vi "FuzzyEx Tanks with PI control.vi"() -> ()   [LabVIEW 2023]
doc: "This example simulates a two-tank system with a fuzzy controller. The system is two tanks of water with a small orifice between the tanks at the bottom of both (height = 0 m). The second tank has another small orifice at the tank bottom that empties into a reservoir at a lower height than the two tanks. The initial properties of the tanks and orifices are shown on the front panel controls below each tank.\n\nThe goal of the simulation is to control the height of tank 2 to the user-specified height setpoint. The control value is the flow rate into tank 1. Therefore, this system is a second-order control system.\n\nThe tanks.fs file represents a fuzzy system with two inputs and one output. The inputs are the height error of tank 2 and the rate of change in height of tank 2. The controller output is the rate of change in flow rate into tank 1."
uses:
  <vilib>/addons/Fuzzy Logic/TypeDefs/FL System.ctl
  <vilib>/addons/Fuzzy Logic/TypeDefs/FL Variable.ctl
  <vilib>/addons/Fuzzy Logic/TypeDefs/FL Membership Function.ctl
  <vilib>/addons/Fuzzy Logic/TypeDefs/FL Membership Function Shape.ctl
  <vilib>/addons/Fuzzy Logic/TypeDefs/FL Rule.ctl
  <vilib>/addons/Fuzzy Logic/TypeDefs/FL Antecedent.ctl
  <vilib>/addons/Fuzzy Logic/TypeDefs/FL Modifier.ctl
  <vilib>/addons/Fuzzy Logic/TypeDefs/FL Antecedent Connective.ctl
  <vilib>/addons/Fuzzy Logic/TypeDefs/FL Consequent.ctl
  <vilib>/addons/Fuzzy Logic/TypeDefs/FL Consequent Implication.ctl
  <vilib>/addons/Fuzzy Logic/TypeDefs/FL Defuzzification.ctl
  <vilib>/addons/Fuzzy Logic/TypeDefs/FL Interpolating polynomials.ctl
  <vilib>/addons/Fuzzy Logic/FL Fuzzy Controller (MISO).vi
  <vilib>/addons/Fuzzy Logic/NI_Fuzzy_Logic_API.lvlib
panel:
  out "fuzzy system out":T1={"input variables"=[{"name"="dH/dT Tank 2", "range"=[-0.01, 0.01, -0.01, 0.01], "MFs"=[{"name"="Fast neg", "shape"=1, "points"=[-0.01, -0.01, -0.006666666666666668, -0.0026666666666666683], "color"=16711680, "user-defined shape index"=0}, {"name"="Slow neg", "shape"=0, "points"=[-0.006666666666666668, -0.0026666666666666683, 0.0], "color"=3342438, "user-defined shape index"=0}, {"name"="Zero", "shape"=0, "points"=[-0.0026666666666666683, 0.0, 0.0026666666666666705], "color"=255, "user-defined shape index"=0}, {"name"="Slow pos", "shape"=0, "points"=[0.0, 0.0026666666666666705, 0.006666666666666665], "color"=16724991, "user-defined shape index"=0}, {"name"="Fast pos", "shape"=1, "points"=[0.0026666666666666705, 0.006666666666666665, 0.01, 0.01], "color"=26214, "user-defined shape index"=0}]}, {"name"="Tank 2 error", "range"=[-0.5, 0.5, -0.5, 0.5], "MFs"=[{"name"="Lg neg", "shape"=1, "points"=[-0.5, -0.5, -0.3, -0.09999999999999998], "color"=16711680, "user-defined shape index"=0}, {"name"="Sm neg", "shape"=0, "points"=[-0.3, -0.09999999999999998, 0.0], "color"=3342438, "user-defined shape index"=0}, {"name"="None", "shape"=0, "points"=[-0.09999999999999998, 0.0, 0.09999999999999998], "color"=16724991, "user-defined shape index"=0}, {"name"="Sm pos", "shape"=0, "points"=[0.0, 0.09999999999999998, 0.30000000000000004], "color"=255, "user-defined shape index"=0}, {"name"="Lg pos", "shape"=1, "points"=[0.09999999999999998, 0.30000000000000004, 0.5, 0.5], "color"=26214, "user-defined shape index"=0}]}], "output variables"=[{"name"="Flow change", "range"=[-0.05, 0.05, -0.05, 0.05], "MFs"=[{"name"="Lg neg", "shape"=0, "points"=[-0.05, -0.05, -0.029999999999999995], "color"=16711680, "user-defined shape index"=0}, {"name"="Med neg", "shape"=0, "points"=[-0.05, -0.029999999999999995, -0.009999999999999993], "color"=3342438, "user-defined shape index"=0}, {"name"="Sm neg", "shape"=0, "points"=[-0.029999999999999995, -0.009999999999999993, 0.0], "color"=16724991, "user-defined shape index"=0}, {"name"="No change", "shape"=0, "points"=[-0.009999999999999993, 0.0, 0.009999999999999976], "color"=255, "user-defined shape index"=0}, {"name"="Sm pos", "shape"=0, "points"=[0.0, 0.009999999999999976, 0.030000000000000016], "color"=10040064, "user-defined shape index"=0}, {"name"="Med pos", "shape"=0, "points"=[0.009999999999999976, 0.030000000000000016, 0.05], "color"=13056, "user-defined shape index"=0}, {"name"="Lg pos", "shape"=0, "points"=[0.030000000000000016, 0.05, 0.05], "color"=26214, "user-defined shape index"=0}]}], "rules"=[{"antecedents"=[{"Var Index"=0, "MF Index"=0, "Cond"=0}, {"Var Index"=1, "MF Index"=0, "Cond"=0}], "antecedent connective"=0, "consequents"=[{"Var Index"=0, "MF Index"=3, "Cond"=0}], "consequent implication"=0, "degree of support"=1.0}, {"antecedents"=[{"Var Index"=0, "MF Index"=0, "Cond"=0}, {"Var Index"=1, "MF Index"=1, "Cond"=0}], "antecedent connective"=0, "consequents"=[{"Var Index"=0, "MF Index"=4, "Cond"=0}], "consequent implication"=0, "degree of support"=1.0}, {"antecedents"=[{"Var Index"=0, "MF Index"=0, "Cond"=0}, {"Var Index"=1, "MF Index"=2, "Cond"=0}], "antecedent connective"=0, "consequents"=[{"Var Index"=0, "MF Index"=5, "Cond"=0}], "consequent implication"=0, "degree of support"=1.0}, {"antecedents"=[{"Var Index"=0, "MF Index"=0, "Cond"=0}, {"Var Index"=1, "MF Index"=3, "Cond"=0}], "antecedent connective"=0, "consequents"=[{"Var Index"=0, "MF Index"=6, "Cond"=0}], "consequent implication"=0, "degree of support"=1.0}, {"antecedents"=[{"Var Index"=0, "MF Index"=0, "Cond"=0}, {"Var Index"=1, "MF Index"=4, "Cond"=0}], "antecedent connective"=0, "consequents"=[{"Var Index"=0, "MF Index"=6, "Cond"=0}], "consequent implication"=0, "degree of support"=1.0}, {"antecedents"=[{"Var Index"=0, "MF Index"=1, "Cond"=0}, {"Var Index"=1, "MF Index"=0, "Cond"=0}], "antecedent connective"=0, "consequents"=[{"Var Index"=0, "MF Index"=2, "Cond"=0}], "consequent implication"=0, "degree of support"=1.0}, {"antecedents"=[{"Var Index"=0, "MF Index"=1, "Cond"=0}, {"Var Index"=1, "MF Index"=1, "Cond"=0}], "antecedent connective"=0, "consequents"=[{"Var Index"=0, "MF Index"=3, "Cond"=0}], "consequent implication"=0, "degree of support"=1.0}, {"antecedents"=[{"Var Index"=0, "MF Index"=1, "Cond"=0}, {"Var Index"=1, "MF Index"=2, "Cond"=0}], "antecedent connective"=0, "consequents"=[{"Var Index"=0, "MF Index"=4, "Cond"=0}], "consequent implication"=0, "degree of support"=1.0}, {"antecedents"=[{"Var Index"=0, "MF Index"=1, "Cond"=0}, {"Var Index"=1, "MF Index"=3, "Cond"=0}], "antecedent connective"=0, "consequents"=[{"Var Index"=0, "MF Index"=5, "Cond"=0}], "consequent implication"=0, "degree of support"=1.0}, {"antecedents"=[{"Var Index"=0, "MF Index"=1, "Cond"=0}, {"Var Index"=1, "MF Index"=4, "Cond"=0}], "antecedent connective"=0, "consequents"=[{"Var Index"=0, "MF Index"=6, "Cond"=0}], "consequent implication"=0, "degree of support"=1.0}, {"antecedents"=[{"Var Index"=0, "MF Index"=2, "Cond"=0}, {"Var Index"=1, "MF Index"=0, "Cond"=0}], "antecedent connective"=0, "consequents"=[{"Var Index"=0, "MF Index"=0, "Cond"=0}], "consequent implication"=0, "degree of support"=1.0}, {"antecedents"=[{"Var Index"=0, "MF Index"=2, "Cond"=0}, {"Var Index"=1, "MF Index"=1, "Cond"=0}], "antecedent connective"=0, "consequents"=[{"Var Index"=0, "MF Index"=2, "Cond"=0}], "consequent implication"=0, "degree of support"=1.0}, {"antecedents"=[{"Var Index"=0, "MF Index"=2, "Cond"=0}, {"Var Index"=1, "MF Index"=2, "Cond"=0}], "antecedent connective"=0, "consequents"=[{"Var Index"=0, "MF Index"=3, "Cond"=0}], "consequent implication"=0, "degree of support"=1.0}, {"antecedents"=[{"Var Index"=0, "MF Index"=2, "Cond"=0}, {"Var Index"=1, "MF Index"=3, "Cond"=0}], "antecedent connective"=0, "consequents"=[{"Var Index"=0, "MF Index"=4, "Cond"=0}], "consequent implication"=0, "degree of support"=1.0}, {"antecedents"=[{"Var Index"=0, "MF Index"=2, "Cond"=0}, {"Var Index"=1, "MF Index"=4, "Cond"=0}], "antecedent connective"=0, "consequents"=[{"Var Index"=0, "MF Index"=6, "Cond"=0}], "consequent implication"=0, "degree of support"=1.0}, {"antecedents"=[{"Var Index"=0, "MF Index"=3, "Cond"=0}, {"Var Index"=1, "MF Index"=0, "Cond"=0}], "antecedent connective"=0, "consequents"=[{"Var Index"=0, "MF Index"=0, "Cond"=0}], "consequent implication"=0, "degree of support"=1.0}, {"antecedents"=[{"Var Index"=0, "MF Index"=3, "Cond"=0}, {"Var Index"=1, "MF Index"=1, "Cond"=0}], "antecedent connective"=0, "consequents"=[{"Var Index"=0, "MF Index"=1, "Cond"=0}], "consequent implication"=0, "degree of support"=1.0}, {"antecedents"=[{"Var Index"=0, "MF Index"=3, "Cond"=0}, {"Var Index"=1, "MF Index"=2, "Cond"=0}], "antecedent connective"=0, "consequents"=[{"Var Index"=0, "MF Index"=2, "Cond"=0}], "consequent implication"=0, "degree of support"=1.0}, {"antecedents"=[{"Var Index"=0, "MF Index"=3, "Cond"=0}, {"Var Index"=1, "MF Index"=3, "Cond"=0}], "antecedent connective"=0, "consequents"=[{"Var Index"=0, "MF Index"=3, "Cond"=0}], "consequent implication"=0, "degree of support"=1.0}, {"antecedents"=[{"Var Index"=0, "MF Index"=3, "Cond"=0}, {"Var Index"=1, "MF Index"=4, "Cond"=0}], "antecedent connective"=0, "consequents"=[{"Var Index"=0, "MF Index"=4, "Cond"=0}], "consequent implication"=0, "degree of support"=1.0}, {"antecedents"=[{"Var Index"=0, "MF Index"=4, "Cond"=0}, {"Var Index"=1, "MF Index"=0, "Cond"=0}], "antecedent connective"=0, "consequents"=[{"Var Index"=0, "MF Index"=0, "Cond"=0}], "consequent implication"=0, "degree of support"=1.0}, {"antecedents"=[{"Var Index"=0, "MF Index"=4, "Cond"=0}, {"Var Index"=1, "MF Index"=1, "Cond"=0}], "antecedent connective"=0, "consequents"=[{"Var Index"=0, "MF Index"=0, "Cond"=0}], "consequent implication"=0, "degree of support"=1.0}, {"antecedents"=[{"Var Index"=0, "MF Index"=4, "Cond"=0}, {"Var Index"=1, "MF Index"=2, "Cond"=0}], "antecedent connective"=0, "consequents"=[{"Var Index"=0, "MF Index"=1, "Cond"=0}], "consequent implication"=0, "degree of support"=1.0}, {"antecedents"=[{"Var Index"=0, "MF Index"=4, "Cond"=0}, {"Var Index"=1, "MF Index"=3, "Cond"=0}], "antecedent connective"=0, "consequents"=[{"Var Index"=0, "MF Index"=2, "Cond"=0}], "consequent implication"=0, "degree of support"=1.0}, {"antecedents"=[{"Var Index"=0, "MF Index"=4, "Cond"=0}, {"Var Index"=1, "MF Index"=4, "Cond"=0}], "antecedent connective"=0, "consequents"=[{"Var Index"=0, "MF Index"=3, "Cond"=0}], "consequent implication"=0, "degree of support"=1.0}], "defuzzification method"=0, "description"="This Fuzzy Logic System file specifies a controller for a tank.", "user MF interpolating polynomials"=[]} {"user MF interpolating polynomials"."coa_x(y) coeff" format="%.4g"; "user MF interpolating polynomials"."Area(y) coeff" format="%.4g"; "user MF interpolating polynomials"."X(y) coeff" format="%.4g"; "user MF interpolating polynomials"."Y(x) coeff" format="%.4g"; "user MF interpolating polynomials"."Y" format="%.4g"; "user MF interpolating polynomials"."X" format="%.4g"; "defuzzification method" items=["Center of Area", "Modified Center of Area", "Center of Sums", "Center of Maximum", "Mean of Maximum"]; "rules"."consequents"."Var Index" min=0; "rules"."consequents"."Cond" items=["=", "!="]; "rules"."consequents"."MF Index" min=0; "rules"."antecedents"."Var Index" min=0; "rules"."antecedents"."Cond" items=["=", "!="]; "rules"."antecedents"."MF Index" min=0; "rules"."consequent implication" items=["Minimum", "Product"]; "rules"."antecedent connective" items=["AND (Minimum)", "AND (Product)", "OR (Maximum)", "OR (Probabilistic)"]; "output variables"."MFs"."shape" items=["Triangle", "Trapezoid", "Singleton", "Sigmoid", "Gaussian", "User-Defined"]; "input variables"."MFs"."shape" items=["Triangle", "Trapezoid", "Singleton", "Sigmoid", "Gaussian", "User-Defined"]}
  out "Valve":bool
  out "Rules Used by Fuzzy Controller":cluster{"Color Box":u32, string}[](array[cluster])
  in  "Stop":bool
  out "Process Monitor":T13(graph)={"h1new"=0.7338316358465902, "h2new"=0.4094942850910191, "y"=0.4126665936635096, "Tank 2 Set Point"=0.5}
  in  "Auto?":bool=TRUE
  out "Tank 2":dbl(slide)=0.4094942850910191 scale=0.0..1.0 scale format="%#.1f"
  in  "Initial Flow":dbl=0.3 min=0.0 max=0.5 step=0.05 format="%.3f"
  in  "Tank 2 Set Point":dbl(slide)=0.2 min=0.0 max=0.5 step=0.01 scale=0.0..0.5
  in  "Time scale factor":dbl=20.0
  out "Simulated dT(s)":dbl=0.021
  in  "Flow Rate In":dbl(knob)=0.4126665936635096 min=0.0 max=0.5 step=0.05 scale=0.0..0.5 scale format="%#.1f"
  out "Orifice 2 Flow Rate":dbl(knob)=0.3538687715086328 min=0.0 max=0.5 step=0.05 scale=0.0..0.5 scale format="%#.1f"
  out "Orifice 1 Flow Rate":dbl(knob)=0.3781382205013306 min=0.0 max=0.5 step=0.05 scale=0.0..0.5 scale format="%#.1f"
  out "Tank 1":dbl(slide)=0.7338316358465902 scale=0.0..1.0 scale format="%#.1f"
  # "Overview: This example simulates a two-tank system with a fuzzy controller.\nInstructions:\n1. Run the VI.\n2. Change the Tank 2 Set Point and see the Fuzzy Logic System Controlling input valve to set the Flow Rate In.\n3. Click Stop to stop the VI."
  # "All rates are in liters/s."
  # "Scroll to the right to see rules"
  # "Change tank level setpoint"
  # "IF"
  # "THEN"
  # "Automatic"
  # "Manual"
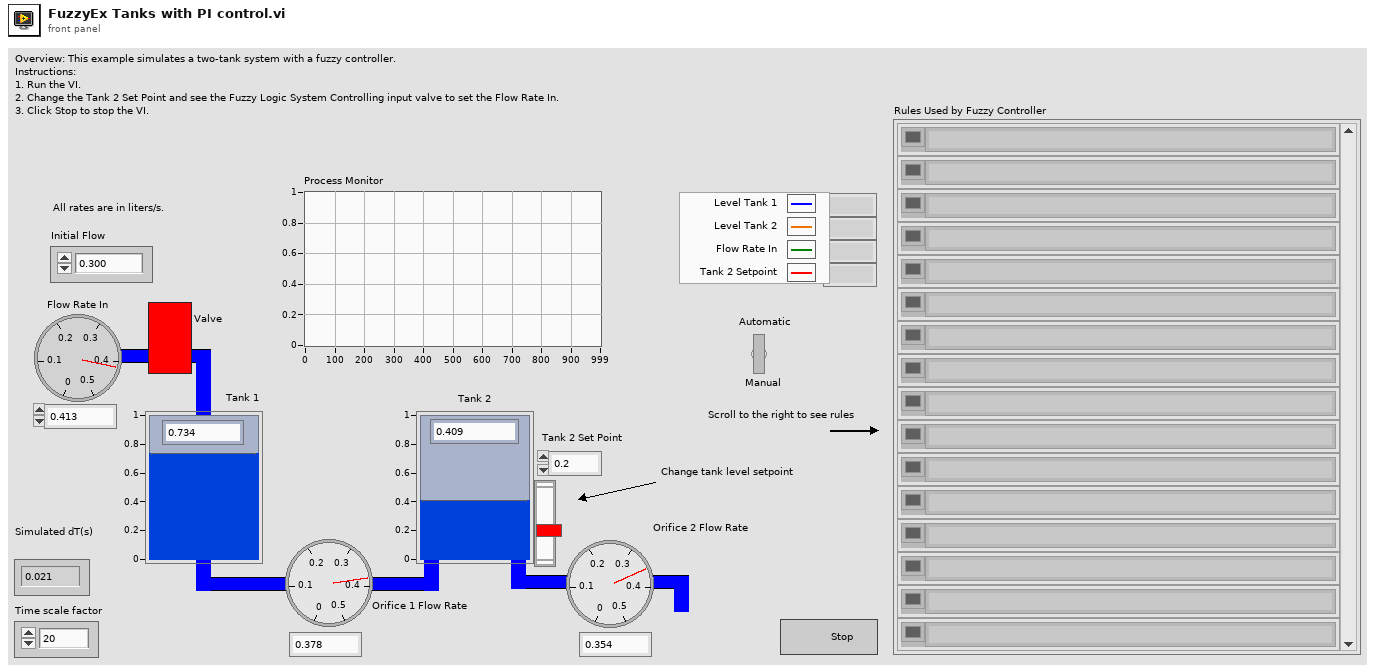
[diagram p1: front panel]
types:
  T1 = typedef "NI_Fuzzy_Logic_API.lvlib/FL System.ctl" = cluster{"input variables":T2[], "output variables":T2[], "rules":T5[], "defuzzification method":T11, "description":string, "user MF interpolating polynomials":T12[]}
  T2 = typedef "NI_Fuzzy_Logic_API.lvlib/FL Variable.ctl" = cluster{"name":string, "range":dbl[], "MFs":T3[]}
  T3 = typedef "NI_Fuzzy_Logic_API.lvlib/FL Membership Function.ctl" = cluster{"name":string, "shape":T4, "points":dbl[], "color":u32, "user-defined shape index":i32}
  T4 = typedef "NI_Fuzzy_Logic_API.lvlib/FL Membership Function Shape.ctl" = u16
  T5 = typedef "NI_Fuzzy_Logic_API.lvlib/FL Rule.ctl" = cluster{"antecedents":T6[], "antecedent connective":T8, "consequents":T9[], "consequent implication":T10, "degree of support":dbl}
  T6 = typedef "NI_Fuzzy_Logic_API.lvlib/FL Antecedent.ctl" = cluster{"Var Index":i32, "MF Index":i32, "Cond":T7}
  T7 = typedef "NI_Fuzzy_Logic_API.lvlib/FL Modifier.ctl" = u16
  T8 = typedef "NI_Fuzzy_Logic_API.lvlib/FL Antecedent Connective.ctl" = u16
  T9 = typedef "NI_Fuzzy_Logic_API.lvlib/FL Consequent.ctl" = cluster{"Var Index":i32, "MF Index":i32, "Cond":T7}
  T10 = typedef "NI_Fuzzy_Logic_API.lvlib/FL Consequent Implication.ctl" = u16
  T11 = typedef "NI_Fuzzy_Logic_API.lvlib/FL Defuzzification.ctl" = u16
  T12 = typedef "NI_Fuzzy_Logic_API.lvlib/FL Interpolating polynomials.ctl" = cluster{"X":dbl[], "Y":dbl[], "Y(x) coeff":dbl[][], "X(y) coeff":dbl[][], "Area(y) coeff":dbl[][], "coa_x(y) coeff":dbl[][]}
  T13 = cluster{"h1new":dbl, "h2new":dbl, "y":dbl, "Tank 2 Set Point":dbl}
  T14 = cluster{"h1new":dbl, "h2new":dbl, "Flow Rate In":dbl, "Tank 2 Set Point":dbl}
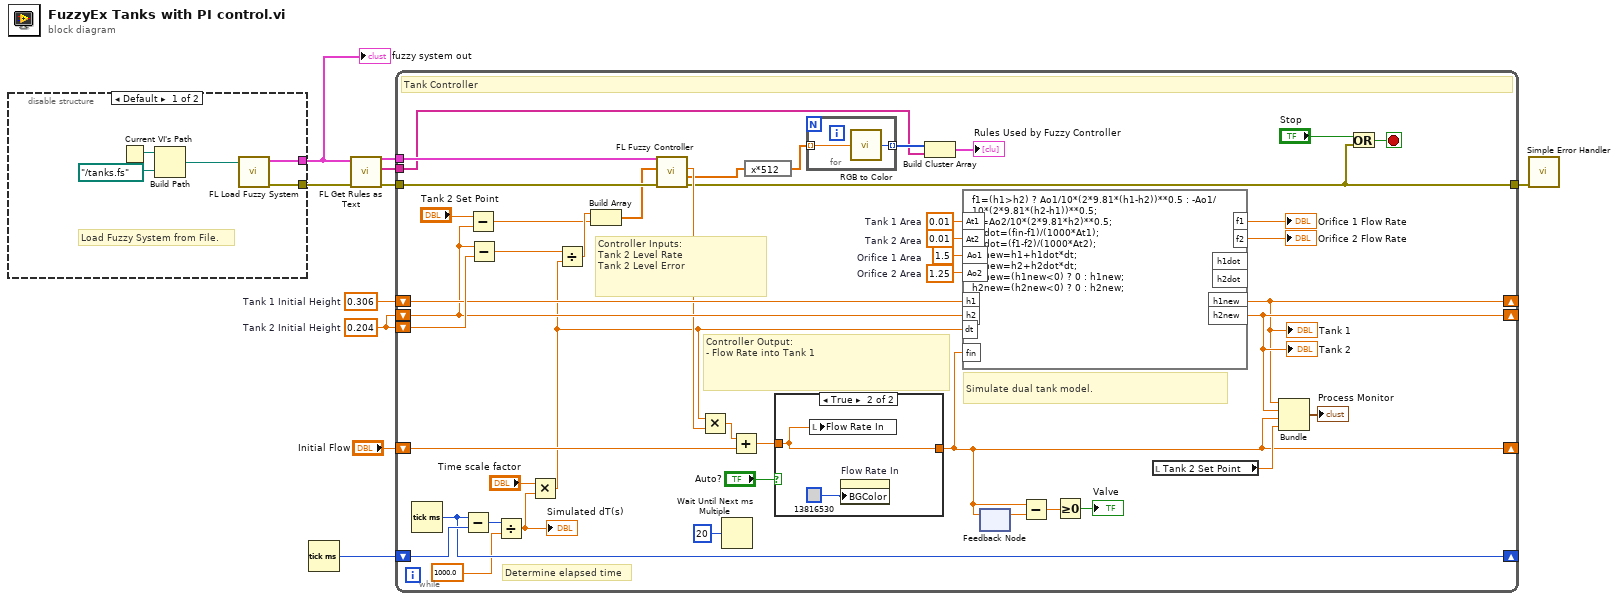
[diagram p0: block diagram]
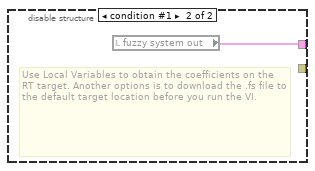
[diagram p2: hidden frame]
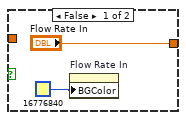
[diagram p3: hidden frame]
diagram:
  w8 = 0.204  # Tank 2 Initial Height
  w7 = 0.306  # Tank 1 Initial Height
  n1 = disable-structure shown="Default" {
    disable-tunnel: [w12 w16] -> w2
    disable-tunnel: [w11 _] -> w1
    frame condition #0 (active) {
      # "Load Fuzzy System from File."
      n2 = Current VI's Path() -> (path=w14:path)
      n3 = Build Path(base path=w14, name or relative path=path "../tanks.fs") -> (appended path=w13:path)
      n4 = call <vilib>:"FL Load Fuzzy System.vi"("file path"=w13) -> ("error out"=w11:errorcluster, "fuzzy system out"=w12:T1)  [unwired: 1 in, 8 out]
    }
    frame condition #1 {
      # "Use Local Variables to obtain the coefficients on the RT target. Another options is to download the .fs file to the default target location before you run the VI."
      n5 = local read "fuzzy system out"() -> (w16:T1)
    }
  }
  "fuzzy system out" <- w2
  n6 = Tick Count (ms)() -> (millisecond timer value=w10:u32)
  n7 = call <vilib>:"FL Get Rules as Text.vi"("error in (no error)"=w1, "fuzzy system in"=w2) -> ("error out"=w4:errorcluster, "rules as text"=w6:string[], "fuzzy system out"=w3:T1)  [unwired: 7 in]
  n8 = while {
    shift-left: w8 -> [w56]
    shift-left: "Initial Flow" -> [w57]
    shift-right: [w23] -> _
    tunnel: w3 -> [w58]
    shift-left: w10 -> [w61]
    shift-right: [w55] -> _
    shift-left: w8 -> [w53]
    shift-right: [w60] -> _
    shift-left: w7 -> [w54]
    shift-right: [w59] -> _
    tunnel: w4 -> [w35]
    tunnel: w6 -> [w19]
    tunnel: [w17] -> w5
    stop <- w18 stop-if-true
    w42 = 1.25  # Orifice 2 Area
    w43 = 1.5  # Orifice 1 Area
    w44 = 0.01  # Tank 2 Area
    w45 = 0.01  # Tank 1 Area
    # "Controller Inputs:\nTank 2 Level Rate\nTank 2 Level Error"
    # "Controller Output:\n- Flow Rate into Tank 1"
    # "Simulate dual tank model."
    # "Determine elapsed time"
    # "Tank Controller"
    n9 = Tick Count (ms)() -> (millisecond timer value=w55:u32)
    n10 = Subtract(x=w55, y=w61) -> (x-y=w36:u32)
    n11 = Subtract(x="Tank 2 Set Point", y=w53) -> (x-y=w31:dbl)
    n12 = Subtract(x=w53, y=w56) -> (x-y=w48:dbl)
    n13 = Divide(x=w36, y=1000.0) -> (x/y=w51:dbl)
    "Simulated dT(s)" <- w51
    n14 = Multiply(x="Time scale factor", y=w51) -> (x*y=w30:dbl)
    n15 = Divide(x=w48, y=w30) -> (x/y=w32:dbl)
    n16 = Build Array(w32, w31) -> (w34:dbl[])
    n17 = call-poly <vilib>:"FL Fuzzy Controller.vi"("error in (no error)"=w35, "input values"=w34, "fuzzy system in"=w58) -> ("error out"=w17:errorcluster, "rule weights"=w28:dbl[], "output value"=w33:dbl)  [unwired: 6 out]
    n18 = Multiply(x=w30, y=w33) -> (x*y=w49:dbl)
    n19 = Wait Until Next ms Multiple(millisecond multiple=u32 20) -> ()  [unwired: 1 out]
    n20 = Add(x=w49, y=w57) -> (x+y=w37:dbl)
    n21 = expression code="x*512"(w28) -> (w27:dbl[])
    n22 = case shown="True" "Auto?" {
      tunnel: ["Flow Rate In" w67] -> w23
      tunnel: w37 -> [_ w67]
      frame False {
        n23 = property on="Flow Rate In" class="Knob (strict)"("BGColor"=u32 16776840) -> ()  [unwired: 2 in, 2 out]
      }
      frame True {
        n24 = local write "Flow Rate In"(w67) -> ()
        n25 = property on="Flow Rate In" class="Knob (strict)"("BGColor"=u32 13816530) -> ()  [unwired: 2 in, 2 out]
      }
    }
    n26 = for {
      tunnel: w27 -> [w62] mode=indexing
      tunnel: [w63] -> w26 mode=indexing
      n27 = call <vilib>:"RGB to Color.vi"("G"=w62) -> ("Color"=w63:u32)  [unwired: 2 in]
    }
    n28 = Build Cluster Array(w26, w19) -> (→"Rules Used by Fuzzy Controller":cluster{"Color":u32, string}[])
    n29 = formula code="f1=(h1>h2) ? Ao1/10*(2*9.81*(h1-h2))**0.5 : -Ao1/10*(2*9.81*(h2-h1))**0.5;\nf2=Ao2/10*(2*9.81*h2)**0.5;\nh1dot=(fin-f1)/(1000*At1);\nh2dot=(f1-f2)/(1000*At2);\nh1new=h1+h1dot*dt;\nh2new=h2+h2dot*dt;\nh1new=(h1new<0) ? 0 : h1new;\nh2new=(h2new<0) ? 0 : h2new;"("fin"=w23, "h1"=w54, "h2"=w53, "At1"=w45, "At2"=w44, "Ao1"=w43, "Ao2"=w42, "dt"=w30) -> ("f1"=→"Orifice 1 Flow Rate":dbl, "f2"=→"Orifice 2 Flow Rate":dbl, "h1new"=w59:dbl, "h2new"=w60:dbl)  [unwired: 2 out]
    "Tank 2" <- w60
    "Tank 1" <- w59
    n30 = feedback-in #1(w23) -> ()
    n31 = feedback #1() -> (w24:dbl)  [unwired: 1 in]
    n32 = Subtract(x=w23, y=w24) -> (x-y=w22:dbl)
    n33 = Greater Or Equal To 0?(x=w22) -> (x >= 0?=→"Valve":bool)
    n34 = local read "Tank 2 Set Point"() -> (w38:dbl)
    n35 = Bundle("h1new"=w59, "h2new"=w60, "Flow Rate In"=w23, "Tank 2 Set Point"=w38) -> (→"Process Monitor":T14)  [unwired: 1 out]
    n36 = Or(x="Stop", y=w17) -> (x .or. y?=w18:bool)
  }
  n37 = call <vilib>:"Simple Error Handler.vi"("error in (no error)"=w5) -> ()  [unwired: 4 in, 5 out]
